vi "FlatToRichcif_manager_QueryInfoRequest.vi"(5 "OutputClusterType":T1, 11 "InputCluster":T3) -> (3 "OutputCluster":T1)   [LabVIEW 2021, in "CIF_Manager_client.lvlib"]
uses:
  cif_manager_QueryInfoRequest_Flat.ctl
  cif_manager_QuerySettings_Flat.ctl
  cif_manager_QueryInfoRequest.ctl
  cif_manager_QuerySettings.ctl
  CIF_Manager_client.lvlib
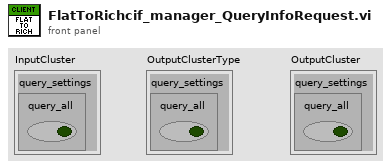
[diagram p1: front panel]
types:
  T1 = typedef "CIF_Manager_client.lvlib/cif_manager_QueryInfoRequest.ctl" = cluster{"query_settings":T2}
  T2 = typedef "CIF_Manager_client.lvlib/cif_manager_QuerySettings.ctl" = cluster{"query_all":bool}
  T3 = typedef "CIF_Manager_client.lvlib/cif_manager_QueryInfoRequest_Flat.ctl" = cluster{"query_settings":T4}
  T4 = typedef "CIF_Manager_client.lvlib/cif_manager_QuerySettings_Flat.ctl" = cluster{"query_all":bool}
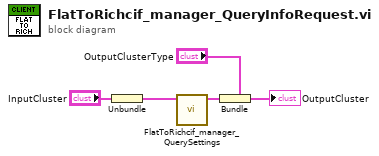
[diagram p0: block diagram]
diagram:
  n1 = Unbundle "Unbundle"("InputCluster") -> ("query_settings"=w2:T4)
  n2 = call "FlatToRichcif_manager_QuerySettings.vi"("InputCluster"=w2) -> ("OutputCluster"=w1:T2)  [unwired: 10 in]
  n3 = Bundle "Bundle"(cluster="OutputClusterType", "query_settings"=w1) -> (→"OutputCluster":T1)
